vi "Contour.vi"   [LabVIEW 2013, in "Advanced Plotting Toolkit.lvlib"]
doc: "Make a contour plot.\n\nThis is a polymorphic VI; you can choose between automatically generating a specific number of contour levels and manually specifying the contour levels you want."
uses:
  Advanced Plotting Toolkit.lvlib
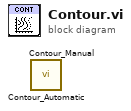
[diagram p0: block diagram]
diagram:
  n1 = call "Contour_Automatic.vi"() -> ()  [unwired: 10 in, 2 out]
  n2 = call "Contour_Manual.vi"() -> ()  [unwired: 10 in, 2 out]
